vi "waitForTermination.vi"(0 "TaskController in":refnum<class "TaskController.lvclass">, 11 "error in (no error)":errorcluster, 12 "timeout[ms]":i32) -> (4 "TaskController out":refnum<class "TaskController.lvclass">, 6 "terminated?":bool, 8 "taskOut":refnum<class "ITask.lvclass">, 10 "taskError":errorcluster, 15 "error out":errorcluster)   [LabVIEW 2023, in "TLC_Daemon.lvlib" / "TaskController.lvclass"]
doc: "Waits for the task termination."
uses:
  TaskController.lvclass
  ITask/ITask.lvclass
  TaskController.lvclass/TaskController.ctl
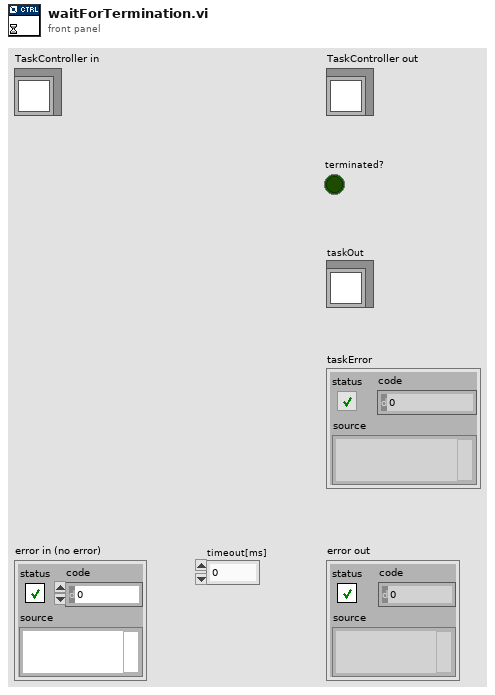
[diagram p1: front panel]
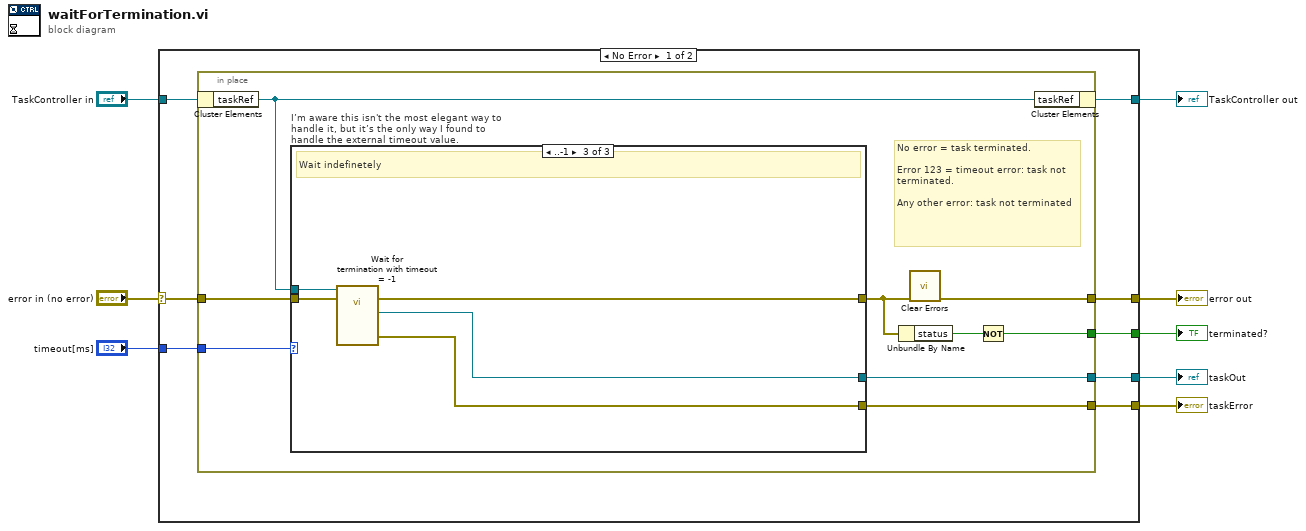
[diagram p0: block diagram]
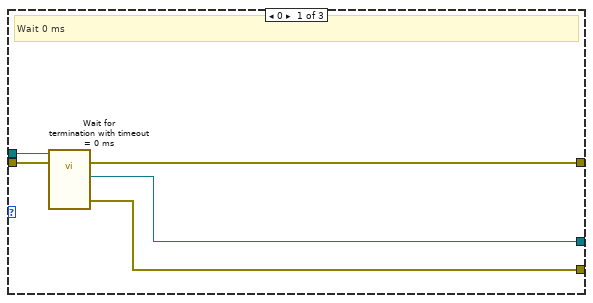
[diagram p2: hidden frame]
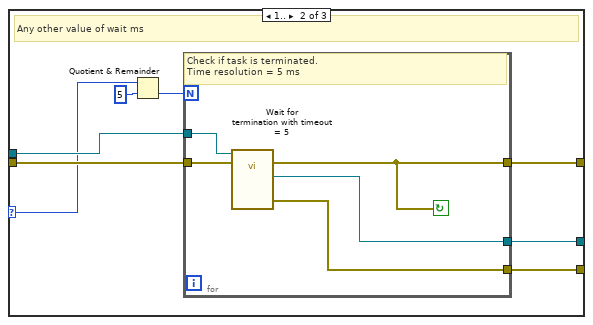
[diagram p3: hidden frame]
diagram:
  n1 = case shown="No Error" "error in (no error)" {
    selector: "error in (no error)" -> [w15 w50]
    tunnel: [w16 w50] -> w7
    tunnel: [w10 w49] -> w5
    tunnel: "TaskController in" -> [w9 w49]
    tunnel: "timeout[ms]" -> [w14 _]
    tunnel: [w13 _] -> w3
    tunnel: [w12 _] -> w2
    tunnel: [w11 _] -> w1
    frame No Error {
      n2 = in-place {
        in-place-border: [w20] -> w16
        in-place-border: w15 -> [w25]
        in-place-border: w14 -> [w24]
        in-place-border: [w19] -> w13
        in-place-border: [w23] -> w12
        in-place-border: [w22] -> w11
        # "No error = task terminated.\n\nError 123 = timeout error: task not terminated.\n\nAny other error: task not terminated"
        n3 = in-place-cluster #1(w9) -> ("taskRef"=w21:refnum<vi>)
        n4 = case "I’m aware this isn't the most elegant way to handle it, but it’s the only way I found to handle the external timeout value." shown="..-1" w24 {
          selector: w24 -> [_ w34 _]
          tunnel: w21 -> [w30 w38 w48]
          tunnel: w25 -> [w29 w37 w47]
          tunnel: [w28 w36 w46] -> w18
          tunnel: [w27 w32 w45] -> w23
          tunnel: [w26 w31 w44] -> w22
          frame 0 {
            # "Wait 0 ms"
            n5 = call-by-ref "Wait for\ntermination with timeout = 0 ms"(reference=w30, error in=w29) -> (error out=w28:errorcluster, 0:"error out"=w26:errorcluster, "ITask out"=w27:refnum<class "ITask.lvclass">)  [unwired: 10 in, 1 out]
          }
          frame 1.. {
            # "Any other value of wait ms"
            n6 = Quotient & Remainder(x=w34, y=5) -> (floor(x/y)=w33:i32)  [unwired: 1 out]
            n7 = for {
              N: w33 -> [_]
              tunnel: w37 -> [w42]
              tunnel: [w41] -> w36
              tunnel: w38 -> [w43]
              tunnel: [w40] -> w32
              tunnel: [w39] -> w31
              stop <- w41 continue-if-true
              # "Check if task is terminated. \nTime resolution = 5 ms"
              n8 = call-by-ref "Wait for\ntermination with timeout = 5"(reference=w43, error in=w42) -> (error out=w41:errorcluster, 0:"error out"=w39:errorcluster, "ITask out"=w40:refnum<class "ITask.lvclass">)  [unwired: 10 in, 1 out]
            }
          }
          frame ..-1 {
            # "Wait indefinetely"
            n9 = call-by-ref "Wait for\ntermination with timeout = -1"(reference=w48, error in=w47) -> (error out=w46:errorcluster, 0:"error out"=w44:errorcluster, "ITask out"=w45:refnum<class "ITask.lvclass">)  [unwired: 10 in, 1 out]
          }
        }
        n10 = Unbundle By Name(w18) -> ("status"=w17:bool)
        n11 = call <vilib>:"Clear Errors.vi"("error in (no error)"=w18) -> ("error out"=w20:errorcluster)  [unwired: 5 in, 1 out]
        n12 = Not(x=w17) -> (.not. x?=w19:bool)
        n13 = in-place-cluster #1("taskRef"=w21) -> (w10:refnum<class "TaskController.lvclass">)
      }
    }
    frame Error {
    }
  }
  "error out" <- w7
  "TaskController out" <- w5
  "terminated?" <- w3
  "taskOut" <- w2
  "taskError" <- w1
